vi "niUSRP EX FSK Rx - 副本.vi"() -> ()   [LabVIEW 2015]
doc: "This example demonstrates demodulation of an FSK signal using devices programmed using the niRFSA driver. This example demonstrates programming techniques for performing FSK deviation measurements and calculating high and low deviations. You can use this example to analyze signals in standards such as Bluetooth.\n\nThe FSK deviation measurements are calculated by first obtaining the raw FSK symbols by removing the oversampled, intra-symbol IQ data points. Then the different frequency symbol values are collected into their respective symbol map 'buckets' and a RMS value is calculated for each symbol map location. Although the values are RMS, which by definition are always positive, the FSK symbol points for negative frequency offsets are negated for clarity purposes only. The output is an array of FSK deviation measurements where the index of the array corresponds directly to the index of the symbol map array contained in the FSK System Parameters cluster. \n\nFor example, if the symbol map array is [-100k, -33k, +33k, +100k] (Hz), the FSK deviation measurements will be reported in an array of four elements with values corresponding to each symbol map values' measured performance, such as [-99.98k, -32.96k, +32.78k, +98.87k] (Hz). These values are for example purposes only."
uses:
  <vilib>/addons/Modulation/Analog/support/mod_Set Error Source.vi
  <vilib>/addons/Modulation/Analog/support/Validators/mod_Fractional Resample Validate.vi
  <vilib>/addons/Modulation/Analog/support/Validators/mod_Check Flush State.vi
  <vilib>/addons/Modulation/Analog/support/mod_FractionalResampler.vi
  <vilib>/addons/Modulation/Analog/support/mod_Integer Rate Interpolation.vi
  <vilib>/addons/Modulation/Analog/support/Validators/mod_Validate Complex Waveform.vi
  <vilib>/addons/Modulation/Analog/support/mod_PerformResampling.vi
  <vilib>/addons/Modulation/Analog/support/Validators/mod_WFErrorHandler.vi
  <vilib>/addons/Modulation/Digital/General/MT Generate FSK System Parameters(M).vi
  <vilib>/addons/Modulation/Digital/Support/Common/Validators/mod_Generate Filter Coefficients Validate.vi
  <vilib>/addons/Modulation/Digital/General/subVIs/mod_Generate Filter Coefficients.vi
  <instrlib>/niUSRP/niUSRP Fetch Rx Data (CDB Cluster).vi
  <vilib>/Utility/error.llb/Error Cluster From Error Code.vi
  <vilib>/addons/Modulation/Analog/support/mod_Resampling Factors.vi
  <vilib>/addons/Modulation/Analog/support/mod_ResamplingFilter.vi
  <vilib>/addons/Modulation/Analog/support/mod_Generate Integer Interpolation Filter.vi
  <vilib>/addons/Modulation/niDMT.lvlib
  <vilib>/addons/Modulation/niAMT.lvlib
panel:
  out "BER":dbl
  in  "number of samples":i64=1000
  in  "Samples Per Symbol":i32=20
  in  "IQ rate":dbl=200000.0 format="%#_6p"
  in  "active antenna":string="RX2"
  out "output bit stream":i8[](array[numeric])=[1, 0, 0, 0, 1, 0, 0, 1, 1, 0, 0, 0, 1, 0, 0, 0, 1, 0, 0, 0, 0, 0, 0, 0, 0, 1, 0, 0, 0, 0, 1, 0, 0, 0, 1, 1, 0, 0, 0, 0, 1, 0, 0, 1, 1, 1, 0, 0]
  in  "device names":refnum<k15>="192.168.10.2"
  in  "Filter Length (symbols)":i32=6
  out "RMS FSK Deviation Measurements (Hz)":dbl[](array[numeric])=[-5290.872047711393, 3325.196765214553] format="%.3p"
  in  "Symbol Phase Continuity":enum16{"continuous", "discontinuous"}(ring)
  in  "Expected  FSK deviation (Hz)":dbl=5000.0 format="%.2p"
  in  "Eye Length, Symbols":i32=3
  in  "Autoscale":bool
  out "Eye Diagram":cluster{"t0":dbl, "dt":dbl, "Y":dbl[]}[](graph)=[{"t0"=9.999999999999972e-06, "dt"=5e-06, "Y"=[-4724.438036616338, -4479.641503778873, -4527.217466105548, -4527.335468398655, -4205.740770407028, -3641.602828019145, -2807.3034745439963, -1834.0951759846917, -1001.8566935773504, -193.57438003707955, 573.07363778137, 990.846736383511, 1219.1298682197591, 1694.8793056816291, 2689.8368536573553, 4210.7603758209225, 5576.024947585654, 6173.6032434453655, 5885.562603638233, 4771.233906834388, 4160.193033332523, 4807.855853479788, 5839.726872710223, 6524.279160168471, 6446.55035280296, 5288.558939212191, 3430.897572918932, 2139.4069922760023, 1712.0369211916461, 1452.8291114098242, 1010.8088117184135, 405.85686862558606, -393.7926469691397, -1484.2027496922071, -2591.2524718833192, -3510.1693885278587, -4093.081585706577, -4472.412744994613, -4832.11042560938, -4866.333404719137, -4654.40429910097, -4711.951205976537, -5313.546414634151, -6304.393274959912, -7153.739850078068, -7554.821180455623, -7536.961311013752, -7181.485752795534, -6608.968234704809, -6081.092914659813, -5706.110689887816, -5226.514271776648, -4895.966653655951, -5152.057497525295, -5890.974042375253, -6419.151494005732, -6402.447252040628, -6274.12174415421, -6158.3430658495345, -5910.2160364824695]}, {"t0"=0.0, "dt"=5e-06, "Y"=[-6158.3430658495345, -5910.2160364824695, -5427.147130947545, -4710.84423276891, -4016.8014148755574, -3544.5889420655776, -3219.8363617027, -2803.5701731071335, -2257.8196701688844, -1816.342629536307, -1603.7044693369205, -1320.5758690884356, -721.2157422085213, -8.880943754301596, 708.7367482422677, 1461.880164210382, 2342.0062746886024, 3290.112458973548, 4047.883487220885, 4474.0358448959605, 4092.5741990119177, 3245.6760099135063, 3192.7151716871704, 4164.641949988062, 5583.711039357467, 6936.316168199011, 7694.157738260012, 6640.106855540738, 4875.076684376678, 5426.386751230875, 7773.294867271847, 9648.984600536513, 9522.23173202106, 7229.47108359629, 5593.98231543865, 6340.3125694995015, 7625.093935066768, 7897.813933446672, 7075.377725310357, 5216.596662740812, 3804.0221817446327, 4051.589050046124, 4925.8974400331435, 5504.150264800366, 5399.213822071406, 4417.460542782094, 2988.6095551874505, 1884.1575556315386, 1349.2354908579048, 1156.4157814980101, 1056.162028644119, 772.6988894476586, 234.5593202711382, -407.3802168472258, -1013.4222378902795, -1674.647925799464, -2491.9611222339136, -3238.7697691745534, -3806.1138949123165, -4262.768646372257, -4535.829633579013]}, {"t0"=-4.999999999999959e-06, "dt"=5e-06, "Y"=[-4262.768646372257, -4535.829633579013, -4599.241087578616, -4499.713968598226, -4526.620124671671, -4916.0559753352945, -5610.85181822579, -6392.0042732329175, -6921.0376472863345, -7183.194016300156, -7089.04731238603, -6582.786211669094, -6025.415544908887, -5491.002100225341, -4868.42328341744, -4282.246004391088, -4065.9272580158267, -4214.04541589411, -4421.023890136324, -4624.926995305612, -4652.451871021729, -4603.477141691125, -4654.906997581185, -4692.17370311602, -4783.846353774806, -4894.819197799572, -4971.074318271915, -5051.1898634741565, -5081.0415131072195, -5028.896762577125, -5070.765280895538, -5151.516640242195, -5021.269783766513, -4869.289875858667, -5114.876727406155, -6140.634538098086, -7540.326136548021, -8439.953228573913, -8697.610470762915, -8514.87958511738, -7882.900903844102, -6935.2362229140435, -5927.629352207114, -5028.782387659598, -4518.594939608156, -4437.008814510093, -4543.336993401064, -4454.4942825191165, -3796.815450517533, -2809.3447122587604, -1786.2963310083098, -848.0079334669327, -83.60943056882071, 553.4912564328394, 909.4489351607899, 1335.4530395924974, 2181.311902226229, 3454.2452634780693, 5420.791693290293, 7453.317411323089, 8510.297037250231, 7724.862379208989]}, {"t0"=-4.999999999999905e-06, "dt"=5e-06, "Y"=[8510.297037250231, 7724.862379208989, 5714.904248577623, 5222.912856093105, 6542.492424869852, 7515.986421560735, 7330.459086427798, 6009.217185294034, 3895.725720791419, 2448.9628984843202, 2180.7175938059568, 2158.1343891893534, 1889.8219884549264, 1258.159032778243, 355.709582023368, -575.4725601770715, -1526.1749531375658, -2482.846427923075, -3374.5529670600386, -4242.456160911923, -4934.951559866785, -5208.230127008767, -5079.301441924647, -4884.8873074368785, -4863.137333743033, -5163.843892988241, -6005.432643318909, -6937.036241857923, -7427.3984647098205, -7687.699728230066, -7657.004643883434, -7192.349844455563, -6551.503621443126, -5826.2821272587125, -5112.973524975087, -4683.895863000425, -4499.148222839919, -4484.291084830834, -4520.635137638361, -4642.869346706426, -4942.65063949015, -5059.035565650833, -5075.744149698536, -5128.762185535445, -5112.660346419432, -5213.942629344681, -5364.480612580232, -5411.091092863799, -5416.516047107908, -5369.224738697783, -5177.990384764717, -4868.285507681264, -4622.810074361489, -4524.8909371366835, -4761.989933875064, -5720.514498949086, -6976.185285283028, -7605.80008789096, -7633.189243734643, -7432.746198670891, -7018.429436707332, -6510.736301011458]}, {"t0"=-4.9999999999998505e-06, "dt"=5e-06, "Y"=[-7018.429436707332, -6510.736301011458, -5883.494240156029, -5106.900828534517, -4522.968681805544, -4189.525733050316, -4029.2644202293227, -3761.6256613445303, -3224.5837544473743, -2657.4718246810294, -1905.6921432302988, -1093.7304437169626, -517.309609652374, -51.293870997626286, 519.2578264147912, 1242.1193540566621, 2074.2457617042573, 3154.548931005476, 4553.637620180563, 6049.012091997126, 7132.671777094343, 6633.67886258513, 4980.894465561312, 4875.012241046783, 6693.128796504307, 8388.060112987241, 8566.756935977652, 6988.362645908198, 4676.220785228258, 3350.424562446264, 3063.0486079282123, 2835.3155736085496, 2375.091865928615, 1574.1252233022344, 624.9751413923816, -372.3932220663811, -1492.69386724596, -2619.7474058706966, -3699.0168062954976, -4538.830288032953, -5141.0679171375, -5591.929848058764, -5773.312125905403, -5727.659918934688, -5512.453854772419, -5533.405507093037, -6339.145864624688, -7485.965658048139, -7982.577349040059, -8007.594612789322, -8054.927756346607, -7680.855238470257, -6759.550765914487, -5841.979327888661, -5162.264108479858, -4582.414056281928, -4154.233106997526, -3977.843998557698, -4103.743480741214, -4520.701081129061, -4930.576343280004, -5118.933588143425]}, {"t0"=-4.999999999999796e-06, "dt"=5e-06, "Y"=[-4930.576343280004, -5118.933588143425, -5234.742825575139, -5275.983184212884, -5191.957302913543, -5201.795391947955, -5182.404691058293, -5004.8461024771705, -4816.465680597025, -4681.0191420866695, -4647.1444974495835, -4582.7876885493315, -4266.463788066646, -3979.4688987279487, -3910.1363598439284, -4029.310609664357, -4469.169972430885, -4955.431564487763, -5218.232157812864, -5329.483016923779, -5386.741760668194, -5401.023050127248, -5472.972798604147, -5538.636052161056, -5284.288960212292, -4860.1954335454175, -4524.139195183586, -4301.709544555951, -4157.581453433255, -3956.633446866387, -3844.7331299332986, -4009.83292405027, -4411.144757137116, -4934.950262353838, -5273.291621566998, -5384.238327247539, -5454.640533040212, -5603.386860007125, -5733.719664868815, -5651.562418313714, -5554.116548668456, -5495.710696358502, -5240.823022892941, -4792.703666461406, -4429.241860779723, -4318.715902171902, -4396.407616612661, -4599.980202589546, -4984.560019440514, -5464.06278893031, -5781.603326438217, -5912.4699263525945, -6054.467940170868, -6086.833862292604, -6087.6490627277935, -6081.373982417588, -5752.882079741344, -5233.118651453003, -4783.473447150784, -4471.457470663375, -4321.654564241531, -4284.495094390014]}, {"t0"=-4.999999999999742e-06, "dt"=5e-06, "Y"=[-4321.654564241531, -4284.495094390014, -4243.083128845192, -4364.627066988062, -4803.82500727497, -5330.1743209421975, -5570.528251632526, -5569.773906037689, -5598.819111672582, -5626.007118459247, -5565.313293669647, -5277.017252401238, -4915.483740320127, -4703.61969132369, -4529.5227969446205, -4392.84764795564, -4217.769892304918, -3956.1622450126747, -3890.5218157123136, -4055.0394938561185, -4336.3236679045895, -4796.750032833973, -5133.447754452825, -5154.570343897508, -5297.699325946998, -5550.990278650009, -5614.498031819818, -5523.197091096859, -5224.73656407081, -4955.316625562237, -4772.423726849531, -4418.051539965465, -4122.472688329127, -4068.1587057135534, -4032.293603501921, -4128.112185323739, -4566.497230215768, -4931.234003002467, -5069.335804043193, -5180.399701921645, -5295.288500561006, -5386.569368244237, -5375.6761866218185, -5226.791245008143, -5065.286473361214, -4989.657938712425, -4873.924279692569, -4756.193317603234, -4660.740566320572, -4493.1113449658515, -4284.731111515527, -4381.0512976081845, -5038.806444990355, -5870.041582289056, -6675.5379462800365, -7463.247517746353, -7983.439170101579, -8140.517308395361, -7892.4058251935985, -7222.296035143907, -6315.887902765867, -5576.765087504833]}, {"t0"=-4.999999999999688e-06, "dt"=5e-06, "Y"=[-6315.887902765867, -5576.765087504833, -5162.775304344052, -5144.763206496177, -5556.980065150696, -5821.265080472366, -5430.588926461716, -4623.508042552064, -3818.3534530364273, -2974.505860773204, -1877.4281429994805, -791.5880613046058, 82.76172481757071, 1055.6897672852338, 2096.0893390913816, 2644.602918731903, 2526.4189207605164, 2656.5629048645296, 3752.203498501529, 5676.3859979455265, 7841.908791527438, 9091.723557835558, 8017.075434648197, 5687.579439036034, 5184.4413718422, 6406.936962280564, 7198.928302021101, 6824.403972596684, 5520.486368687506, 3551.618113047714, 1999.6350732730853, 1497.23715409971, 1175.039581604048, 615.3583863957425, -16.3218226392551, -733.2438985795986, -1523.6986297934936, -2225.21653465329, -3135.867303659251, -3998.846098429856, -4308.525357243702, -4428.622353785205, -4506.439230198759, -4586.155703543308, -5289.979987591934, -6441.307447187701, -7193.660985319492, -7583.931068102672, -7713.376306383106, -7461.631787371195, -6911.445762853932, -6242.934662076033, -5630.9479547657165, -5079.189754108816, -4685.465536940872, -4739.904984601392, -5014.196769137665, -5282.063911329001, -5615.02096438154, -5712.0876417550235, -5668.681651840942, -5786.145102214489]}, {"t0"=-4.999999999999634e-06, "dt"=5e-06, "Y"=[-5668.681651840942, -5786.145102214489, -5903.153327928242, -5753.894053952932, -5363.5892965156, -5088.488647675327, -4970.066957502859, -4826.508297810927, -4659.726121598623, -4370.283840711408, -4087.0173321331763, -4165.889156814342, -4602.50411779792, -5207.799084440001, -5715.9581140754, -5809.588250304393, -5685.087360644126, -5641.6780073238015, -5553.410336279632, -5333.064552623476, -5033.872803243529, -4713.629837879203, -4509.662542827022, -4366.640373433996, -4147.753124319223, -3911.8692330437043, -3743.706259772996, -3751.2139665546015, -3844.5942611928585, -4110.950406386994, -4690.788617416749, -5237.7075402788405, -5531.9935972179, -5970.585339132254, -6554.923519061652, -6638.540405718727, -6395.284628504931, -6145.633991531834, -5671.82110166184, -5190.687861688652, -5081.979499843246, -5386.675911159556, -6078.5009129628925, -6614.95560519527, -6562.434451972911, -6092.024120225586, -5423.618798722659, -4722.516029557213, -3942.3726229711724, -2902.1411232411333, -1788.255802250907, -939.7814137924937, -25.11744029574739, 1160.7756376655568, 2393.1739268445044, 3391.647501724722, 3917.6529984614117, 3664.986120177738, 2993.2516234726477, 3312.4432128112553, 4957.514059199095, 6633.14704348343]}, {"t0"=-4.9999999999995794e-06, "dt"=5e-06, "Y"=[4957.514059199095, 6633.14704348343, 7185.209685105235, 6233.102534701634, 4579.10120764255, 4098.010892838069, 4740.887647242038, 5317.471804476632, 5550.222967208677, 5323.788360917638, 4519.724855134173, 2965.525027947785, 1365.7635789654134, 347.6292871544979, -345.53068558125415, -951.4684394226093, -1649.3069702741234, -2359.8459834445725, -2931.0438555190435, -3433.2946263379886, -3854.2211513369057, -4495.567049447335, -5681.17685555336, -6790.530243801868, -7335.707407913596, -7503.327335851196, -7364.233740539694, -6951.351578785753, -6402.063414035826, -5947.346871809158, -5542.211980651732, -5019.6554705720455, -4734.91206200093, -5015.746774267752, -5431.735107699769, -5537.860223203794, -5455.337720039489, -5376.142774036401, -5285.784149338847, -4870.862388069521, -4376.3422431823, -4292.404297610411, -4305.246761435874, -4116.958943043513, -3942.699240764231, -3911.739509654282, -3792.6196910745266, -3641.278019425166, -3683.6454555921127, -4051.639627869279, -4729.931461921644, -5431.71982717472, -5986.742268094931, -6556.303421307482, -7236.047529062158, -7494.261000493484, -7176.317174158201, -6831.239076594963, -6459.863367406298, -5965.263068214916, -5550.342206498837, -5502.475249003641]}, {"t0"=-4.999999999999525e-06, "dt"=5e-06, "Y"=[-5550.342206498837, -5502.475249003641, -5972.792087910679, -6371.066515370097, -6291.272314567246, -6080.486892047455, -5650.988813792576, -4793.387165959974, -3822.8502514050138, -2798.042747452945, -1947.2751110998872, -1232.6391605343888, -366.8613315146726, 532.0275637245887, 1572.540773374869, 2635.521760291023, 3326.7324297077075, 3334.914659566371, 2872.7520186555416, 2742.206455861426, 3265.1762296511865, 4392.943320511714, 5791.46679258194, 6720.356844751742, 6790.606178611998, 5673.415360742786, 4221.85523914082, 4384.008028163667, 5883.437866973693, 7013.772401025282, 7208.2837016097055, 6178.775060509371, 4735.912867808703, 4765.195210742718, 6142.9434430983665, 7439.848262351225, 7961.205049859501, 6823.90844513157, 4904.818375349904, 5021.441568987202, 6765.582070351731, 7987.174059737578, 8050.938138067237, 6827.266230341797, 4846.878951396014, 3689.8822880756256, 3685.5374668231843, 3917.1126561725955, 4109.734634896469, 3981.9426041193547, 3290.442475863753, 2283.53367047461, 1276.3717447714243, 360.8327964728609, -394.2920990209828, -1001.210204046781, -1644.6468107684834, -2460.6665292335942, -3266.902799306858, -3959.917553379072, -4614.263821715514, -5282.195506216171]}, {"t0"=-4.999999999999471e-06, "dt"=5e-06, "Y"=[-4614.263821715514, -5282.195506216171, -6026.494684140296, -6608.050182565815, -6871.394088638881, -6960.147305985516, -6761.7499689527685, -6167.774494753619, -5568.238228098808, -5363.394650787003, -5691.191893907084, -6444.205064766062, -6996.595847190284, -7113.244673677802, -7057.530717760587, -6808.272575346182, -6462.180981670981, -6055.523854410122, -5457.604521071934, -4914.242070942525, -4534.379548090716, -4187.876939232803, -3885.741276825479, -3714.3246052830973, -3783.669867695837, -4091.6741078442833, -4642.626020586017, -5231.480776791795, -5522.549624509722, -5558.683607977223, -5606.054132460306, -5724.461634271828, -5751.373317401883, -5563.12530887274, -5284.537614300493, -5015.2271229778635, -4708.010332021176, -4394.513128868018, -4081.094859187602, -3829.7160081809197, -3803.1557814730913, -4021.1868246208846, -4135.670157929671, -4168.118984320529, -4609.931203988711, -5026.9823107619995, -4971.135139474579, -4990.177473234478, -5236.50296801762, -5424.00493352496, -5440.208262238011, -5316.1033629267295, -5245.068258140205, -5066.073050397125, -4697.46489285073, -4553.504083306527, -4888.054193939877, -5813.105940228509, -6839.6349759580535, -7391.3673468449715, -7660.976144772664, -7644.987555521]}, {"t0"=-4.999999999999417e-06, "dt"=5e-06, "Y"=[-7660.976144772664, -7644.987555521, -7287.498792625413, -6658.831718178556, -5870.275458589557, -5070.555826944818, -4252.488806963298, -3667.5169110257857, -3281.005982588891, -2586.719027402859, -1770.4043877300646, -1175.8393765472363, -517.7545365300944, 230.89280906895468, 1043.962152362203, 2148.189727614108, 3499.275700409513, 5020.68274154634, 6229.2830855831835, 6624.0558367052145, 5617.2924784850375, 4093.2334567940384, 4423.2482384162, 6015.2091980334435, 6903.731707030129, 6686.251295127893, 5360.572695394452, 3754.3992349484997, 3081.657506556695, 3019.3915238151476, 2860.4230204425444, 2561.56409754009, 2169.1221201614158, 1566.4425962650375, 551.3657977589526, -614.1470776496149, -1533.991164481682, -2372.016275708854, -3320.768471192135, -4253.201793307267, -4912.564591105957, -5270.479400922661, -5515.617011572414, -5629.716081402764, -5500.476236167782, -5264.75252969468, -5111.8355856847, -5062.245228380783, -5341.808080213805, -6140.804987054622, -6914.041109532217, -7186.56495110989, -7138.436703703578, -7022.0273964459275, -6729.099286954071, -6112.755546600173, -5493.106493558151, -5048.496888500124, -4865.532830517098, -5255.585354470429, -5954.861473663697, -6374.543061404588]}]
  in  "M-FSK":i32=2
  in  "Symbol Rate, Hz":dbl=10000.0 format="%.2p"
  in  "Gain":dbl=10.0
  in  "Tx Filter BT":dbl=0.5 format="%.2f"
  in  "TX Filter":T1(ring)=enum."Raised Cosine"
  out "error out":errorcluster caption="Error Out"
  in  "stop":bool
  in  "Number of Symbols":i32=1000
  in  "Carrier Frequency, Hz":dbl=467450000.0 format="%.2p"
  # "Device"
  # "Acquisition"
  # "Measured Deviation"
  # "Modulation"
  # "For a reliable lock, we recommend a minimum Number of Symbols of 20 * M-FSK."
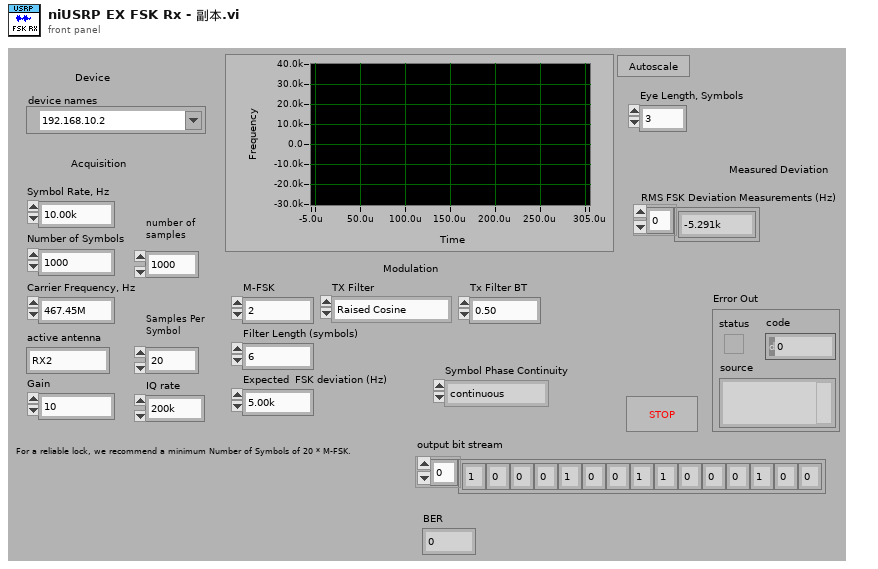
[diagram p1: front panel]
types:
  T1 = enum16{"none", "Raised Cosine", "Root Raised Cos", "Gaussian"}
  T2 = enum16{"FSK", "PSK", "QAM", "MSK", "PAM", "ASK", "CPM"}
  T3 = cluster{"samples per symbol (16)":i32, "symbol map":dbl[], "symbol phase continuity":enum16{"continuous", "discontinuous"}}
  T4 = typedef "niAMT.lvlib/Complex Data Waveform.ctl" = cluster{"t0":dbl, "dt":dbl, "Y":cdb[]}
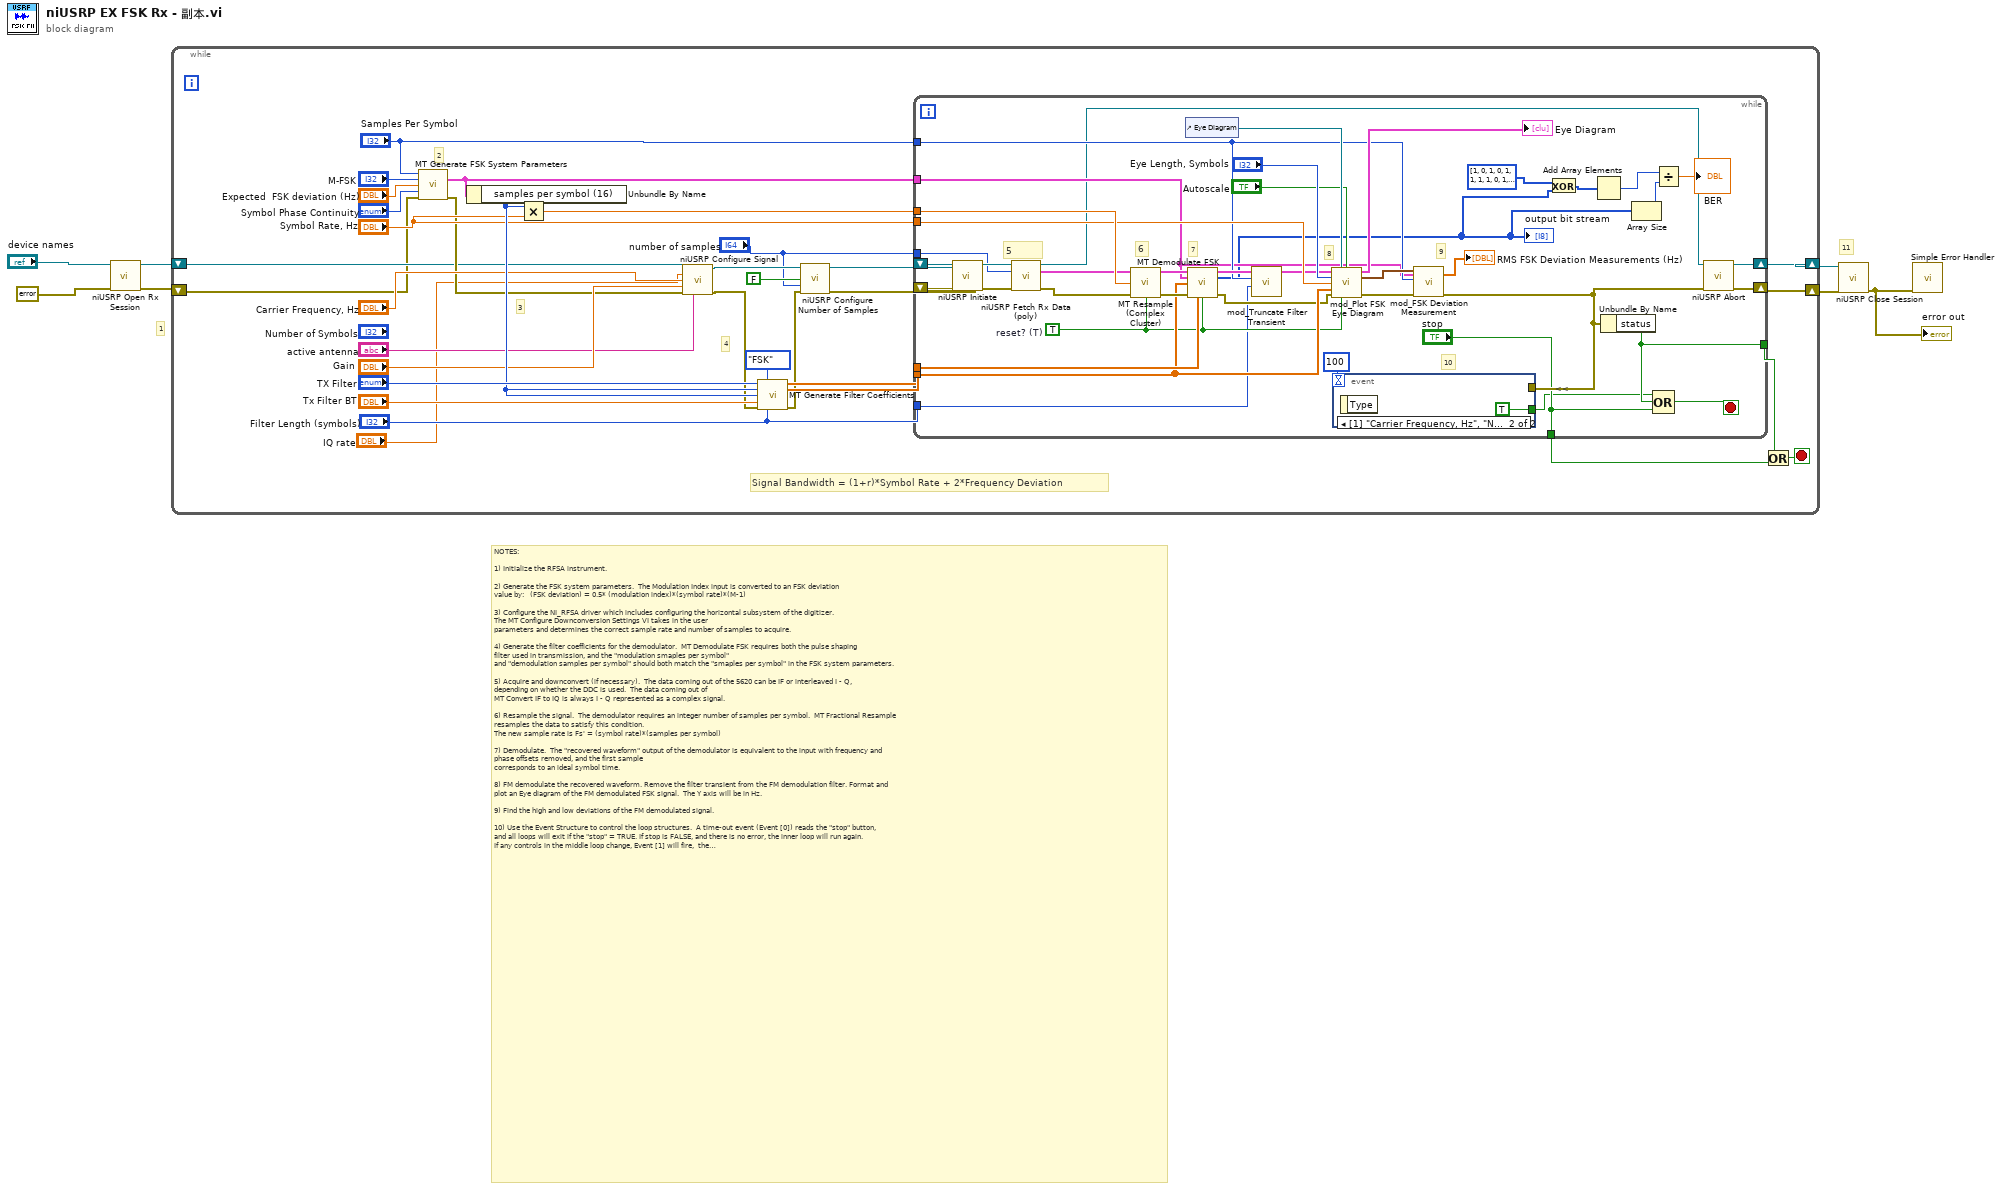
[diagram p0: block diagram]
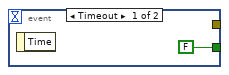
[diagram p2: hidden frame]
diagram:
  # "11"
  # "1"
  # "NOTES:\n\n1) Initialize the RFSA instrument. \n\n2) Generate the FSK system parameters.  The Modulation Index input is converted to an FSK deviation \nvalue by:   (FSK deviation) = 0.5* (modulation index)*(symbol rate)*(M-1)\n\n3) Configure the NI_RFSA driver which includes configuring the horizontal subsystem of the digitizer.  \nThe MT Configure Downconversion Settings VI takes in the user \nparameters and determines the correct sample rate and number of samples to acquire.\n\n4) Generate the filter coefficients for the demodulator.  MT Demodulate FSK requires both the pulse shaping \nfilter used in transmission, and the \"modulation smaples per symbol\" \nand \"demodulation samples per symbol\" should both match the \"smaples per symbol\" in the FSK system parameters. \n\n5) Acquire and downconvert (if necessary).  The data coming out of the 5620 can be IF or interleaved I - Q, \ndepending on whether the DDC is used.  The data coming out of \nMT Convert IF to IQ is always I - Q represented as a complex signal.\n\n6) Resample the signal.  The demodulator requires an integer number of samples per symbol.  MT Fractional Resample \nresamples the data to satisfy this condition.  \nThe new sample rate is Fs' = (symbol rate)*(samples per symbol)\n\n7) Demodulate.  The \"recovered waveform\" output of the demodulator is equivalent to the input with frequency and \nphase offsets removed, and the first sample \ncorresponds to an ideal symbol time.\n\n8) FM demodulate the recovered waveform. Remove the filter transient from the FM demodulation filter. Format and \nplot an Eye diagram of the FM demodulated FSK signal.  The Y axis will be in Hz.\n\n9) Find the high and low deviations of the FM demodulated signal.\n\n10) Use the Event Structure to control the loop structures.  A time-out event (Event [0]) reads the \"stop\" button, \nand all loops will exit if the \"stop\" = TRUE. If stop is FALSE, and there is no error, the inner loop will run again.  \nIf any controls in the middle loop change, Event [1] will fire,  the inner loop will exit, and the middle loop will run again.  \nIf any controls in the outer loop change, Event [2] will fire, both the inner and middle loops will exit, and the outer \nloop will run again.\n\n11) If the middle loop exits, the instrument handles and the receiver info will be closed."
  n1 = call <instrlib>:"niUSRP Open Rx Session.vi"("device names"="device names", "error in (no error)"=errorcluster {"status"=FALSE, "code"=0, "source"=""} ("error out")) -> ("session handle out"=w3:refnum<k15>, "error out"=w1:errorcluster)  [unwired: 12 in]
  n2 = while {
    shift-right: [w13] -> w6
    shift-left: w3 -> [w12]
    shift-right: [w25] -> w5
    shift-left: w1 -> [w11]
    stop <- w40 stop-if-true
    # "Signal Bandwidth = (1+r)*Symbol Rate + 2*Frequency Deviation"
    # "4"
    # "3"
    # "2"
    n3 = call-poly <vilib>:"MT Generate FSK System Parameters.vi"("samples per symbol (16)"="Samples Per Symbol", "M-FSK (2)"="M-FSK", "FSK deviation (Hz)"="Expected  FSK deviation (Hz)", "symbol phase continuity"="Symbol Phase Continuity", "error in (no error)"=w11) -> ("FSK system parameters"=w34:T3, "error out"=w16:errorcluster)  [unwired: 9 out]
    n4 = Unbundle By Name(w34) -> ("samples per symbol (16)"=w26:i32)
    n5 = Multiply(x=w26, y="Symbol Rate, Hz") -> (x*y=w29:dbl)
    n6 = call <instrlib>:"niUSRP Configure Signal.vi"("session handle"=w12, "IQ rate"="IQ rate", "carrier frequency"="Carrier Frequency, Hz", "gain"="Gain", "error in (no error)"=w16, "active antenna"="active antenna") -> ("session handle out"=w14:refnum<k15>, "error out"=w15:errorcluster)  [unwired: 5 in, 3 out]
    n7 = call <vilib>:"MT Generate Filter Coefficients.vi"("pulse shaping filter (none)"="TX Filter", "modulation type"=T2."FSK", "pulse shaping samples per symbol (16)"=w26, "matched samples per symbol (16)"=w26, "filter parameter"="Tx Filter BT", "error in (no error)"=w15, "filter length (symbols)"="Filter Length (symbols)") -> ("pulse shaping filter coefficients"=w35:dbl[], "matched filter coefficients"=w36:dbl[], "error out"=w27:errorcluster)  [unwired: 6 out]
    n8 = call <instrlib>:"niUSRP Configure Number of Samples.vi"("session handle"=w14, "number of samples is finite"=FALSE, "number of samples"="number of samples", "error in (no error)"=w27) -> ("session handle out"=w23:refnum<k15>, "error out"=w24:errorcluster)  [unwired: 10 in]
    n9 = while {
      tunnel: ["stop"] -> w39
      tunnel: [w76] -> w38
      tunnel: w36 -> [w73]
      tunnel: w34 -> [w61]
      tunnel: w29 -> [w80]
      tunnel: w35 -> [w77]
      tunnel: "Symbol Rate, Hz" -> [w74]
      tunnel: "Samples Per Symbol" -> [w63]
      tunnel: "Filter Length (symbols)" -> [w62]
      shift-right: [w53] -> w13
      shift-left: w23 -> [w56]
      shift-right: [w52] -> w25
      shift-left: w24 -> [w58]
      tunnel: "number of samples" -> [w47]
      stop <- w81 stop-if-true
      w70 = TRUE  # reset? (T)
      # "10"
      # "9"
      # "8"
      # "7"
      # "6"
      # "5"
      # "<<"
      n10 = call <instrlib>:"niUSRP Initiate.vi"("session handle"=w56, "error in (no error)"=w58) -> ("session handle out"=w55:refnum<k15>, "error out"=w57:errorcluster)  [unwired: 12 in]
      n11 = call-poly <instrlib>:"niUSRP Fetch Rx Data (poly).vi"("session handle"=w55, "number of samples"=w47, "error in (no error)"=w57) -> ("session handle out"=w51:refnum<k15>, "data"=w59:cluster{"t0":dbl, "dt":dbl, "Y":cdb[]}, "error out"=w54:errorcluster)  [unwired: 9 in, 1 out]
      n12 = call <vilib>:"MT Resample (Complex Cluster).vi"("input complex waveform"=w59, "desired sample rate (Hz)"=w80, "error in (no error)"=w54, "reset? (T)"=w70) -> ("output complex waveform"=w79:T4, "error out"=w78:errorcluster)  [unwired: 2 in, 8 out]
      n13 = control-ref of="Eye Diagram"() -> (w72:refnum<vi>)
      n14 = call <vilib>:"MT Demodulate FSK.vi"("input complex waveform"=w79, "FSK system parameters"=w61, "matched filter coefficients"=w73, "error in (no error)"=w78, "pulse shaping filter coefficients"=w77, "reset? (T)"=w70) -> ("recovered complex waveform"=w66:T4, "output bit stream"=w44:i8[], "error out"=w64:errorcluster)  [unwired: 1 in, 6 out]
      "output bit stream" <- w44
      n15 = call <vilib>:"mod_Truncate Filter Transient.vi"("filter length (sym)"=w62, "samples/symbol"=w63, "input complex waveform"=w66) -> ("output complex waveform"=w65:T4)  [unwired: 8 out]
      n16 = call <vilib>:"mod_Plot FSK Eye Diagram.vi"("Input Complex Waveform"=w65, "Rx Eye Diagram"=w72, "autoscale"="Autoscale", "eye length"="Eye Length, Symbols", "Symbol Rate, Hz"=w74, "matched filter coefficients"=w73, "error in (no error)"=w64, "Reset?"=w70) -> ("FSK Eye Diagram"=→"Eye Diagram":cluster{"t0":dbl, "dt":dbl, "Y":dbl[]}[], "output FM demodulated waveform"=w68:waveform(dbl), "error out"=w67:errorcluster)  [unwired: 5 out]
      n17 = call <vilib>:"mod_FSK Deviation Measurement.vi"("FM demodulated waveform in"=w68, "FSK system parameters"=w61, "samples per symbol (16)"=w63, "error in (no error)"=w67) -> ("RMS FSK Deviation Measurements (Hz)"=→"RMS FSK Deviation Measurements (Hz)":dbl[], "error out"=w50:errorcluster)  [unwired: 14 out]
      n18 = event shown="[1] \"Carrier Frequency, Hz\", \"Number of Symbols\", \"TX Filter\", \"Tx Filter BT\", \"M-FSK\", \"Gain\", \"Symbol Rate, Hz\": 值改变" {
        selector: _ -> [_ _]
        dyn-events: _ -> [_ _]
        timeout: 100 -> [_ _]
        tunnel: [FALSE ("stop") TRUE ("stop")] -> w48
        tunnel: w50 -> [_ _]
        event Timeout {
          n19 = event-data() -> ()  [unwired: 2 out]
        }
        event "Carrier Frequency, Hz", "Number of Symbols", "TX Filter", "Tx Filter BT", "M-FSK", "Gain", "Symbol Rate, Hz": Value Change {
          n20 = event-data() -> ()  [unwired: 2 out]
        }
      }
      n21 = Exclusive Or(1:w44, 2:i8[] [1, 0, 1, 0, 1, 1, 1, 1, 0, 1, 0, 0, 0, 0, 1, 0, 1, 1, 0, 1, 1, 0, 1, 0, 1, 1, 0, 0, 1, 1, 1, 0, 1, 1, 1, 1, 1, 0, 0, 0, 0, 1, 1, 0, 0, 1, 1, 0, 0, 0, 1, 0, 1, 0, 0, 1, 1, 1, 1, 0, 0, 0, 0, 1, 0, 1, 0, 1, 1, 1, 1, 0, 0, 1, 0, 0, 1, 1, 0, 1, 1, 1, 0, 0, 1, 1, 1, 0, 1, 1, 0, 1, 0, 0, 1, 0, 0, 0, 1, 0, 0, 1, 1, 1, 0, 0, 0, 0, 1, 0, 1, 0, 0, 0, 1, 1, 1, 0, 1, 0, 1, 0, 0, 0, 0, 1, 0, 0, 1, 0, 0, 0, 0, 1, 1, 0, 0, 0, 1, 1, 0, 0, 0, 1, 0, 0, 0, 0, 0, 0, 1, 0, 0, 0, 0, 0, 1, 0, 1, 0, 1, 0, 1, 1, 1, 1, 0, 1, 1, 0, 0, 0, 0, 1, 1, 0, 0, 1, 0, 0, 1, 0, 0, 1, 0, 1, 0, 0, 0, 1, 1, 1, 1, 1, 1, 0, 0, 0, 0, 0, 1, 0, 1, 0, 0, 1, 0, 1, 0, 1, 0, 0, 0, 0, 0, 0, 1, 1, 1, 0, 0, 0, 0, 1, 1, 1, 1, 0, 0, 0, 0, 1, 1, 1, 1, 1, 1, 0, 1, 1, 0, 1, 1, 1, 1, 0, 0, 0, 1, 0, 1, 0, 1, 0, 1, 1, 1, 1, 1, 0, 1, 0, 0, 0, 0, 0, 1, 1, 0, 1, 0, 0, 1, 1, 1, 1, 0, 1, 1, 1, 0, 0, 0, 0, 0, 1, 0, 1, 0, 0, 1, 1, 0, 0, 1, 1, 1, 1, 1, 0, 1, 0, 1, 1, 1, 0, 0, 0, 0, 0, 1, 0, 0, 0, 0, 0, 0, 1, 1, 0, 1, 0, 0, 1, 0, 1, 1, 1, 1, 0, 1, 0, 1, 0, 0, 0, 1, 0, 1, 0, 0, 1, 0, 0, 0, 1, 0, 0, 0, 0, 0, 0, 1, 0, 1, 1, 1, 0, 1, 1, 0, 1, 1, 1, 1, 1, 1, 0, 1, 1, 1, 1, 0, 0, 1, 1, 1, 1, 0, 1, 0, 0, 0, 0, 0, 0, 0, 1, 1, 1, 0, 0, 1, 1, 0, 1, 1, 0, 0, 1, 1, 0, 1, 1, 1, 1, 0, 1, 1, 0, 1, 0, 1, 0, 0, 1, 1, 0, 1, 1, 0, 0, 1, 1, 1, 1, 0, 0, 0, 1, 0, 1, 0, 0, 0, 1, 1, 1, 0, 1, 1, 1, 1, 1, 0, 0, 0, 0, 1, 0, 0, 0, 0, 1, 0, 1, 0, 0, 0, 0, 1, 0, 0, 1, 0, 1, 1, 0, 1, 0, 0, 0, 1, 0, 1, 0, 1, 0, 1, 1, 0, 1, 1, 1, 1, 0, 1, 0, 0, 0, 0, 0, 0, 1, 1, 1, 0, 0, 0, 0, 1, 1, 1, 0, 0, 1, 0, 1, 1, 0, 1, 1, 0, 0, 1, 0, 0, 0, 1, 0, 1, 1, 1, 0, 1, 0, 0, 1, 1, 1, 0, 1, 0, 0, 0, 0, 1, 1, 0, 1, 1, 0, 1, 1, 1, 1, 1, 1, 1, 1, 0, 1, 0, 1, 0, 0, 1, 1, 1, 1, 0, 0, 0, 0, 1, 0, 1, 1, 0, 1, 0, 0, 1, 1, 1, 0, 0, 1, 0, 1, 1, 1, 1, 1, 1, 1, 1, 1, 0, 1, 1, 1, 1, 1, 1, 0, 0, 1, 1, 0, 1, 1, 0, 0, 1, 1, 0, 1, 0, 0, 0, 0, 0, 1, 0, 0, 1, 1, 0, 1, 0, 1, 0, 0, 0, 1, 1, 1, 1, 0, 0, 1, 1, 0, 0, 0, 0, 0, 0, 1, 1, 1, 1, 1, 0, 1, 0, 1, 0, 1, 1, 1, 1, 0, 0, 0, 1, 0, 1, 1, 1, 1, 0, 0, 1, 1, 1, 1, 0, 0, 0, 0, 0, 0, 1, 0, 1, 1, 1, 0, 0, 0, 0, 1, 1, 1, 1, 1, 0, 0, 0, 0, 1, 0, 1, 0, 1, 1, 1, 0, 1, 1, 0, 0, 1, 0, 0, 1, 0, 0, 1, 1, 0, 0, 1, 0, 1, 0, 0, 1, 1, 0, 0, 1, 0, 1, 0, 1, 0, 1, 1, 1, 0, 0, 1, 0, 0, 0, 1, 0, 0, 1, 0, 1, 1, 0, 1, 1, 1, 1, 0, 0, 1, 1, 0, 0, 1, 1, 1, 1, 1, 1, 1, 0, 1, 0, 0, 0, 1, 1, 1, 0, 0, 0, 1, 1, 1, 0, 0, 1, 1, 1, 0, 0, 0, 0, 1, 1, 0, 1, 0, 1, 1, 0, 1, 0, 1, 1, 1, 1, 0, 0, 1, 0, 0, 1, 0, 1, 1, 0, 1, 0, 0, 0, 1, 0, 0, 1, 1, 1, 1, 0, 1, 1, 0, 0, 1, 1, 1, 1, 0, 1, 1, 0, 0, 0, 1, 0, 1, 1, 1, 0, 0, 0, 0, 0, 0, 0, 0, 0, 0, 0, 1, 1, 0, 0, 0, 0, 1, 1, 0, 0, 0, 0, 1, 0, 0, 1, 0, 1, 1, 0, 0, 1, 0, 0, 1, 1, 0, 0, 1, 0, 0, 0, 1, 1, 1, 1, 0, 0, 1, 1, 1, 0, 1, 0, 0, 0, 0, 1, 1, 1, 1, 1, 0, 1, 1, 0, 1, 0, 1, 1, 1, 1, 1, 0, 0, 1, 1, 0, 1, 0, 1, 0, 0, 0, 0, 0, 0, 0, 1, 0, 1, 1, 1, 1, 0, 0, 1, 0, 1, 0, 1, 0, 1, 0, 0, 1, 0, 0, 1, 1, 1, 0, 1, 1, 1, 0, 0, 1, 1, 0, 0, 1, 1, 1, 1, 0, 0, 1, 1, 1, 1, 0, 0, 1, 0, 0, 1, 0, 0, 1, 1, 0, 1, 1, 1, 1, 0, 1, 0, 0, 1, 1, 1, 0, 0, 1, 1, 0, 0, 1, 0, 1, 0, 0, 1, 1, 0, 1, 1, 0, 1, 0, 1, 0, 1, 0, 1, 0, 0, 1, 0, 0] ("数组")) -> (0:w45:i8[])
      n22 = Add Array Elements(numeric array=w45) -> (sum=w42:i8)
      n23 = Unbundle By Name(w50) -> ("status"=w76:bool)
      n24 = Array Size(array=w44) -> (size(s)=w43:i32)
      n25 = Compound Arithmetic op=OR(w48, w76, "stop") -> (w81:bool)
      n26 = Divide(x=w42, y=w43) -> (x/y=→"BER":dbl)
      n27 = call <instrlib>:"niUSRP Abort.vi"("session handle"=w51, "error in (no error)"=w50) -> ("session handle out"=w53:refnum<k15>, "error out"=w52:errorcluster)  [unwired: 12 in]
    }
    n28 = Or(x=w38, y=w39) -> (x .or. y?=w40:bool)
  }
  n29 = call <instrlib>:"niUSRP Close Session.vi"("session handle"=w6, "error in (no error)"=w5) -> ("error out"=w7:errorcluster)  [unwired: 13 in]
  "error out" <- w7
  n30 = call <vilib>:"Simple Error Handler.vi"("error in (no error)"=w7) -> ()  [unwired: 1 in, 8 out]
